vi "UI_AutoRefresh_Do.vi"(8 "error in (no error)":errorcluster, 9 "Parameters":T1={"Write TipStrips with details (T)"=TRUE, "Write Captions with UserLabels (T)"=TRUE, "Mode (ind only)"=enum."Indicators only", "Enable nested stream (T)"=TRUE}, 10 "Databox_sealed":refnum<class "Databox_sealed.lvclass">, 11 "UIA_ChildTestMaster in":refnum<class "UIA_UTsupport.lvclass">) -> (0 "error out":errorcluster, 3 "UIA_ChildTestMaster out":refnum<class "UIA_UTsupport.lvclass">)   [LabVIEW 2020, in "UIA_UTsupport.lvlib" / "UIA_UTsupport.lvclass"]
doc: "Enable nested stream : Permet le routage de la databox vers les nested UIA de l'acteur. On peut couper ce ruissellement si les nested n'ont pas besoin de databox pour optimiser le programme."
uses:
  UIA_UTsupport.lvclass
  D:/Projets/STEP AT/UI Actor/UI_Actor/UI_Actor/UI_Actor.lvclass
  UI_Actor/UI_Actor/ctl_AR_Parameters.ctl
  UI_Actor/UI_Actor/ctl_AR_Mode.ctl
  support/Databox.lvlibp/Databox_sealed/Databox_sealed.lvclass
  gloglo.vi
  UI_Actor/UI_Actor/UI_Actor.lvclass
  support/Databox.lvlibp/TypesTools/Data/Data.lvclass
  D:/Projets/STEP AT/UI Actor/support/Actor Framework.lvlibp/1abvi3w/vi.lib/ActorFramework/Actor/Actor.lvclass
  D:/Projets/STEP AT/UI Actor/tests/UIA_UTsupport/UIA_UTsupport.lvclass
panel:
  out "DIM SysLabels":string[](array[string])
  out "Latest Data":dbl[](array[numeric])
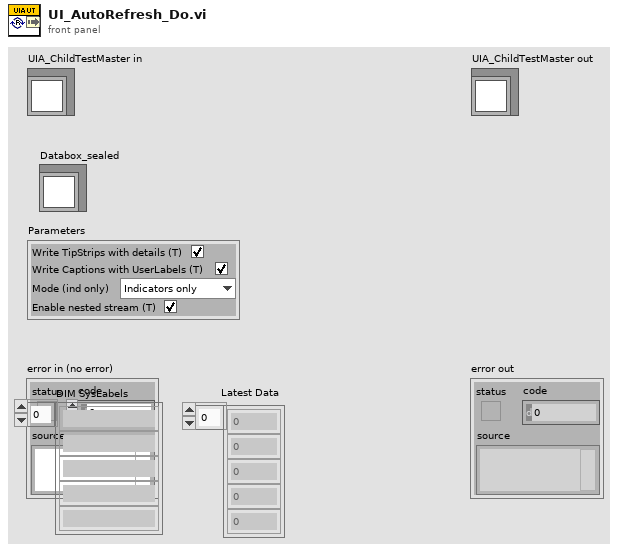
[diagram p1: front panel]
types:
  T1 = typedef "UI_Actor.lvlib/UI_Actor.lvclass/ctl_AR_Parameters.ctl" = cluster{"Write TipStrips with details (T)":bool, "Write Captions with UserLabels (T)":bool, "Mode (ind only)":T2, "Enable nested stream (T)":bool}
  T2 = typedef "UI_Actor.lvlib/UI_Actor.lvclass/ctl_AR_Mode.ctl" = enum16{"Controls only", "Indicators only", "All"}
  T3 = typedef "UI_Actor.lvlib/UI_Actor.lvclass/ctl_InternalMapItem.ctl" = cluster{"Config":refnum<class "Config.lvclass">, "LatestData":refnum<class "Data.lvclass">}
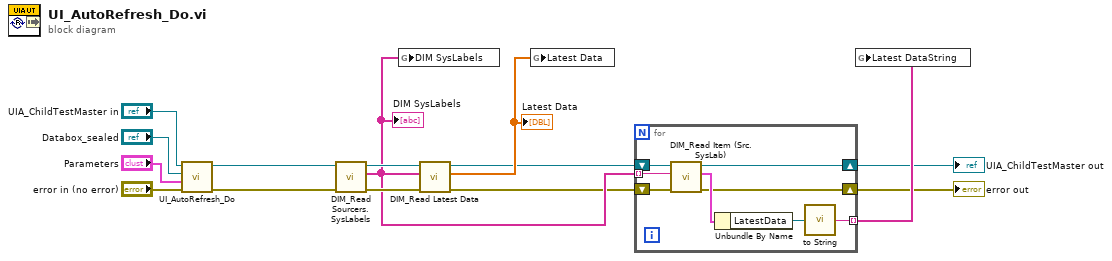
[diagram p0: block diagram]
diagram:
  n1 = call-parent "UI_AutoRefresh_Do.vi"("error in (no error)"="error in (no error)", "Parameters"="Parameters", "Databox_sealed"="Databox_sealed", "UI_Actor in"="UIA_ChildTestMaster in") -> ("error out"=w8:errorcluster, "UI_Actor out"=w9:refnum<class "UIA_UTsupport.lvclass">)  [unwired: 6 in]
  n2 = call "DIM_Read Sourcers.SysLabels.vi"("error in (no error)"=w8, "UI_Actor in"=w9) -> ("error out"=w10:errorcluster, "DIM Sourcer.SysLabels"=w6:string[], "UI_Actor out"=w11:refnum<class "UIA_UTsupport.lvclass">)  [unwired: 7 in]
  "DIM SysLabels" <- w6
  n3 = global write "gloglo.vi" "DIM SysLabels"(w6) -> ()
  n4 = call "DIM_Read Latest Data.vi"("error in (no error)"=w10, "Src.SysLabels"=w6, "UI_Actor in"=w11) -> ("error out"=w2:errorcluster, "Latest Data"=w7:dbl[], "UI_Actor out"=w4:refnum<class "UIA_UTsupport.lvclass">)  [unwired: 6 in]
  "Latest Data" <- w7
  n5 = global write "gloglo.vi" "Latest Data"(w7) -> ()
  n6 = for {
    tunnel: w6 -> [w23] mode=indexing
    tunnel: [w20] -> w5 mode=indexing
    shift-right: [w17] -> w3
    shift-left: w4 -> [w19]
    shift-right: [w16] -> w1
    shift-left: w2 -> [w18]
    n7 = call "DIM_Read Item (Src.SysLab).vi"("error in (no error)"=w18, "Sourcer.SysLabel"=w23, "UI_Actor in"=w19) -> ("error out"=w16:errorcluster, "DIM Item"=w22:T3, "UI_Actor out"=w17:refnum<class "UIA_UTsupport.lvclass">)  [unwired: 5 in, 1 out]
    n8 = Unbundle By Name(w22) -> ("LatestData"=w21:refnum<class "Data.lvclass">)
    n9 = call "to String.vi"("Data"=w21) -> ("String"=w20:string)
  }
  "error out" <- w1
  "UIA_ChildTestMaster out" <- w3
  n10 = global write "gloglo.vi" "Latest DataString"(w5) -> ()
